vi "Parse State Queue++.vi"(0 "State Queue":string, 1 "Name(\"\" to use uuid)":string, 2 "Response Arguments":string, 7 "Error In (no error)":errorcluster, 9 "Dequeue Timeout(0ms)":i32, 11 "Response Timeout(1000ms)":i32=10000) -> (4 "Remaining States":string, 6 "Current State":string, 8 "Arguments":string, 10 "Argument - State":string, 15 "From Who":string)   [LabVIEW 2014, in "JKI-State-Machine-Plus.lvlib"]
doc: "Parses the JKI State Machine state queue and returns the current state that will execute next with the associated arguments.\n\nFor instructions on how to use the JKI State Machine, examples and video tutorials, visit:\nhttp://jkisoft.com/state-machine/\n\n<B>Inputs:</B>\n <B>State Queue:</B> The entire state queue is wired to this input. This should come from the main JKI State Machine shift register.\n <B>Error In</B> The error cluster from the JKI State Machine is wired to this input. If an error occures and appears on this input, the current state output returns the \"Error Handler\" state.\n\n<B>Outputs:</B>\n <B>Remaining States:</B> Returns all the next states that should execute after the current state completes. These should be passed through the current state in the state machine. These can also be modified or augmented within the current state if necessary.\n <B>Current State:</B> Returns the current state that should execute next in the state machine. If an error is wired to the Error input then the current state output becomes \"Error Handler\".\n <B>Arguments:</B> Returns any argument(s) that may be used in the current state string. These arguments come after the \">>\" characters. <B>Note:</B> The arguments variable must not contain any unprintable characters like linefeed or carriage return.\n\n<B>State Syntax:</B>\nStateCategory: State >> Argument\nLine Terminator: Line feed\n <B>Example:</B>\nUI: Help >> About\n\nWhere \"UI\" is the state category\nWhere \"Help\" is the state\nWhere \"About\" is the argument\n <B>Other Examples:</B>\nApp Data: Initialize\nUI: Initialize\nHelp >> About\n\n<B>Commenting:</B>\nTo add a comment use \"//\" or \"#\" and all text to the right will be ignored\n <B>Commenting Example:</B>\nUI: Initialize // This initializes the UI\n# This whole line is a comment\n// Another comment line\n\nJKI State Machine™ 2018.0.7.45\nhttp://jki.net/state-machine/\nCopyright (C) 2005-2018, JKI <info@jki.net>\nALL RIGHTS RESERVED"
uses:
  JKI-State-Machine-Plus.lvlib
  _Support/_Cross JKI StateMachine State Data.ctl
  _Support/_Cross JKI StateMachine State Response.ctl
  <vilib>/addons/_JKI Toolkits/State Machine/_JKI_lib_State_Machine.llb/Add State(s) to Queue__JKI_lib_State_Machine.vi
  Utility/Build Internal State String.vi
  _Support/_uuid.vi
  _Support/_JKISMQFGV.vi
  <vilib>/regexp/Match Regular Expression.xnode
panel:
  # "For instructions on how to use the JKI State Machine, examples and video tutorials, visit:\nhttp://jki.net/state-machine/\n\nJKI State Machine™\nhttp://jki.net/state-machine/\nCopyright (C) 2005-2017, JKI <info@jki.net>\nALL RIGHTS RESERVED"
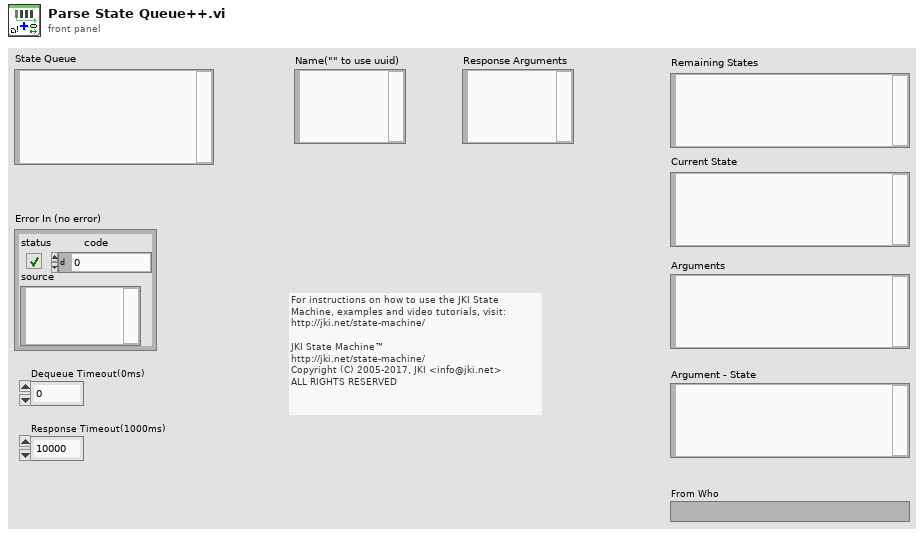
[diagram p1: front panel]
types:
  T1 = typedef "JKI-State-Machine-Plus.lvlib/_Cross JKI StateMachine State Data.ctl" = cluster{"state":string, "args":string, "source":string, "RespQ":refnum<queue>}
  T2 = typedef "JKI-State-Machine-Plus.lvlib/_Cross JKI StateMachine State Response.ctl" = cluster{"error":errorcluster, "Response Data":string}
  T3 = typedef "JKI-State-Machine-Plus.lvlib/_JKISMQ.ctl" = cluster{"Queue":refnum<queue>, "Locked Status":refnum<data-value>, "Stand Alone Mode":bool}
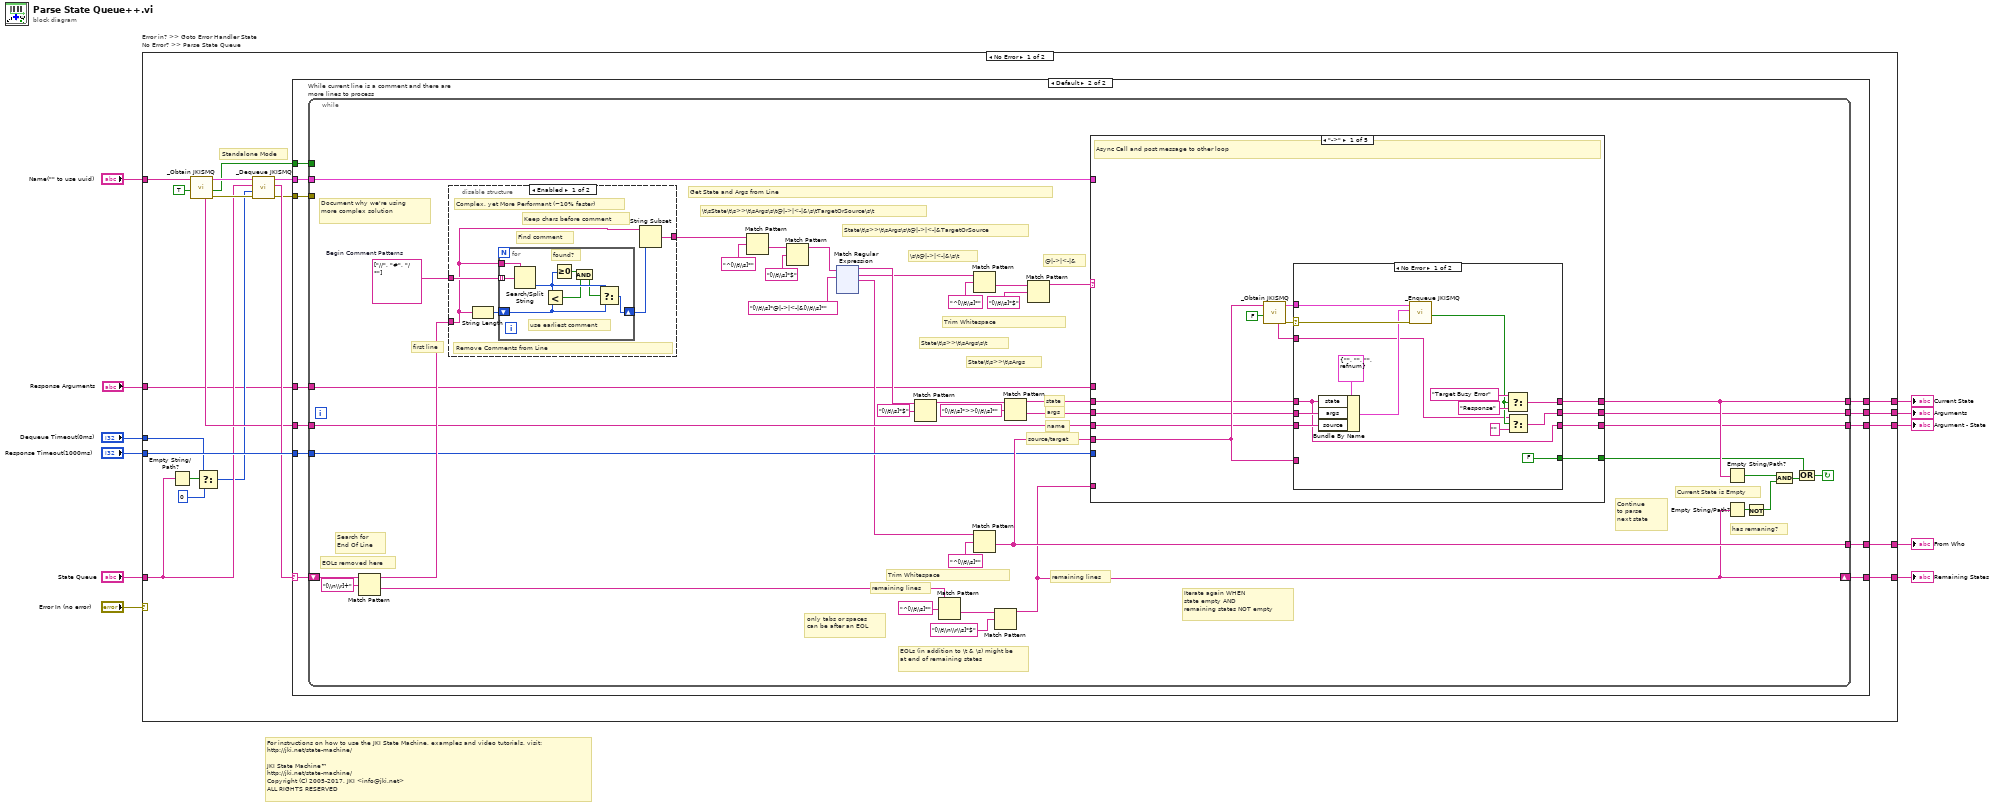
[diagram p0: block diagram]
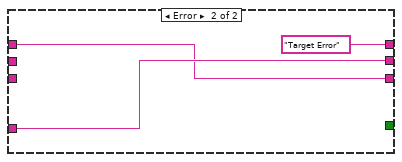
[diagram p3: hidden frame]
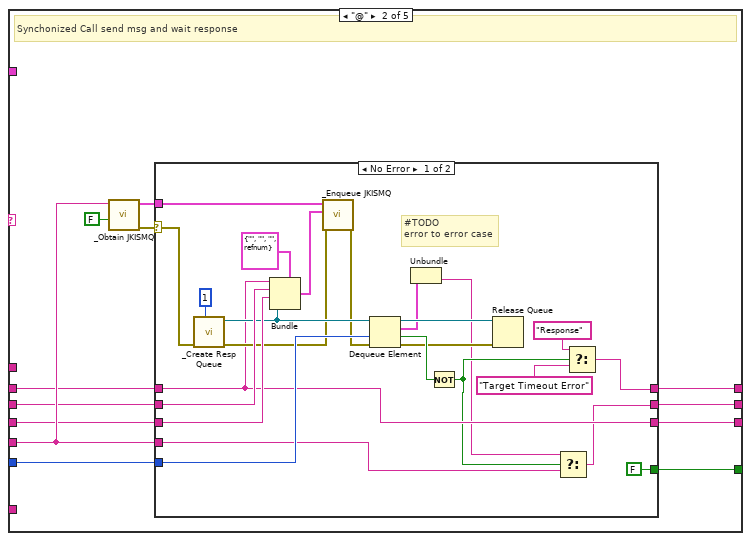
[diagram p4: hidden frame]
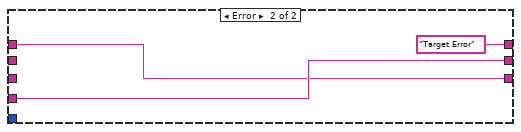
[diagram p5: hidden frame]
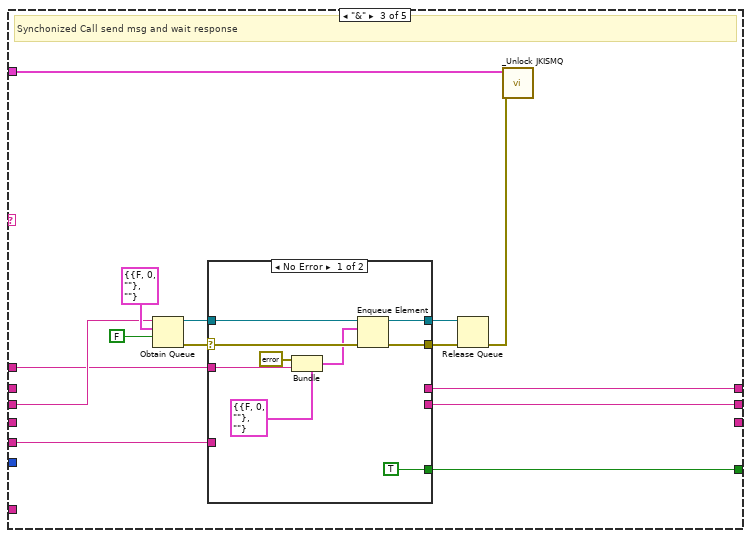
[diagram p6: hidden frame]
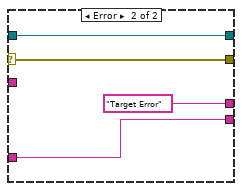
[diagram p7: hidden frame]
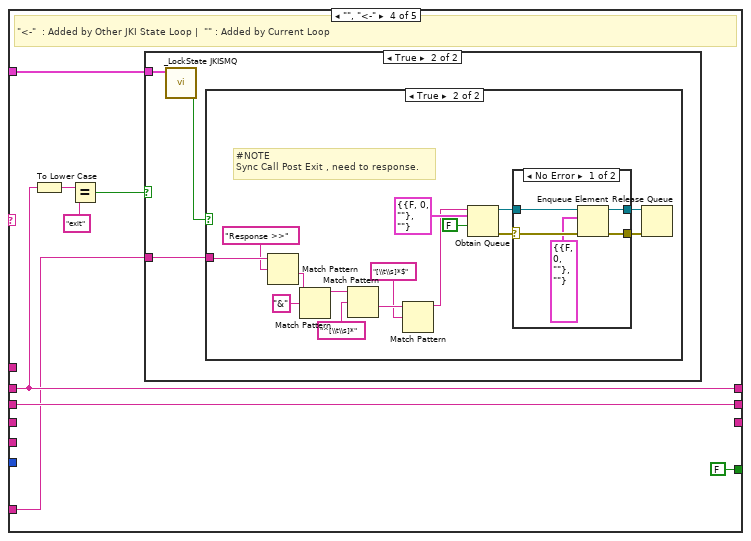
[diagram p8: hidden frame]
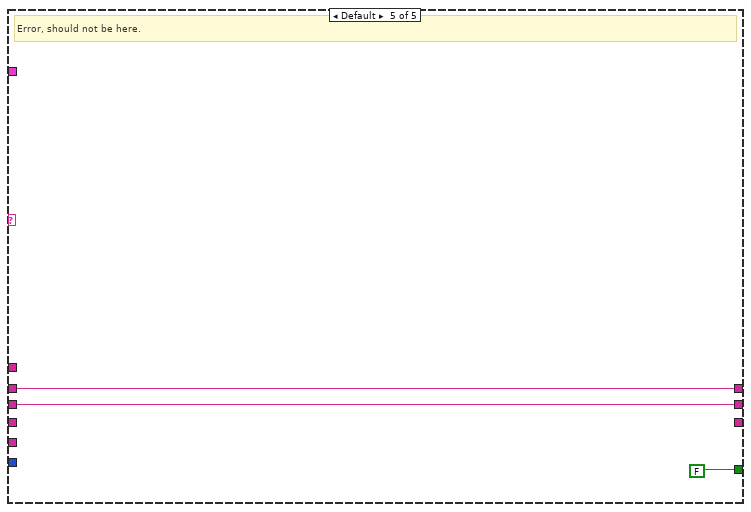
[diagram p12: hidden frame]
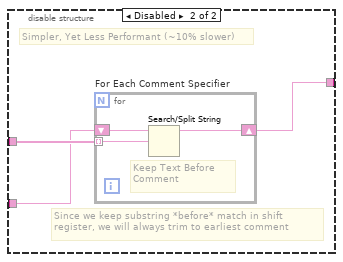
[diagram p13: hidden frame]
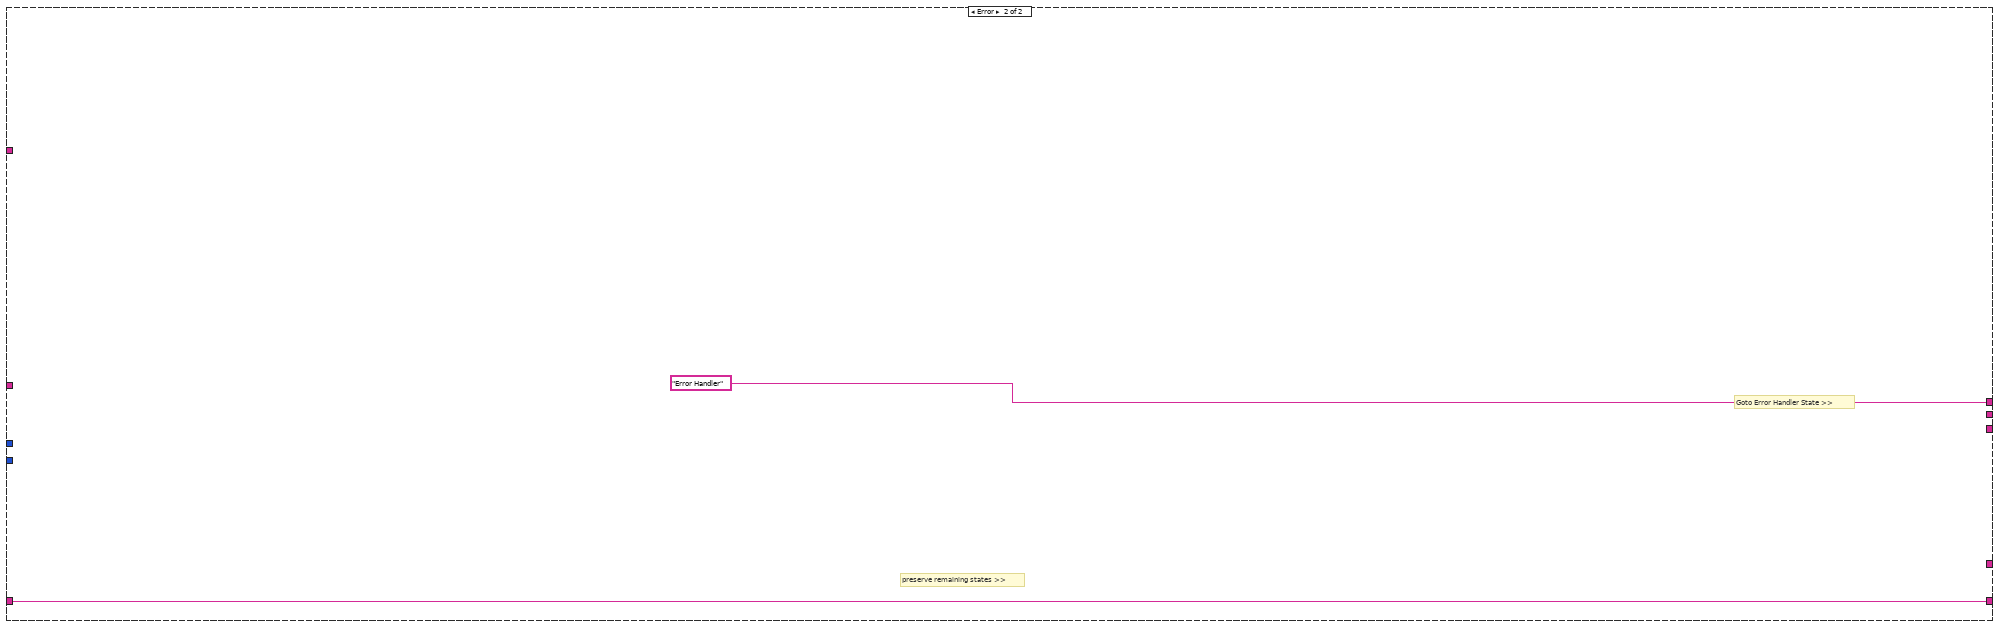
[diagram p14: hidden frame]
diagram:
  # "For instructions on how to use the JKI State Machine, examples and video tutorials, visit:\nhttp://jki.net/state-machine/\n\nJKI State Machine™\nhttp://jki.net/state-machine/\nCopyright (C) 2005-2017, JKI <info@jki.net>\nALL RIGHTS RESERVED"
  n1 = case "Error in? >> Goto Error Handler State\nNo Error? >> Parse State Queue" shown="No Error" "Error In (no error)" {
    tunnel: [w30 w353] -> w11
    tunnel: [w32 "Error Handler"] -> w9
    tunnel: [w31 _] -> w8
    tunnel: "State Queue" -> [w18 w353]
    tunnel: "Response Timeout(1000ms)" -> [w29 _]
    tunnel: "Name(\"\" to use uuid)" -> [w28 _]
    tunnel: [w27 _] -> w4
    tunnel: "Dequeue Timeout(0ms)" -> [w17 _]
    tunnel: [w13 _] -> w2
    tunnel: "Response Arguments" -> [w12 _]
    frame No Error {
      # "Standalone Mode"
      n2 = Empty String/Path?(string/path=w18) -> (empty?=w19:bool)
      n3 = call "_Obtain JKISMQ.vi"("create if not found? (T)"=TRUE, "Name(\"\" to use uuid) in"=w28) -> ("Error out"=w24:errorcluster, "Stand Alone Mode"=w14:bool, "JKISMQ"=w26:T3, "Name"=w21:string)  [unwired: 6 in]
      n4 = Select(t=w17, s=w19, f=0) -> (s? t:f=w15:i32)
      n5 = call "_Dequeue JKISMQ.vi"("Error in"=w24, "Dequeue Timeout(0ms)"=w15, "State(s) in (\"\")"=w18, "JKISMQ"=w26) -> ("Error out"=w20:errorcluster, "States Out"=w22:string, "JKISMQ"=w23:T3)  [unwired: 5 in]
      n6 = case shown="Default" w22 {
        selector: w22 -> [_ w38]
        tunnel: [_ w44] -> w32
        tunnel: [_ w43] -> w31
        tunnel: [_ w42] -> w30
        tunnel: w29 -> [_ w41]
        tunnel: [_ w40] -> w27
        tunnel: w21 -> [_ w39]
        tunnel: w23 -> [_ w37]
        tunnel: w20 -> [_ w36]
        tunnel: w14 -> [_ w35]
        tunnel: [_ w34] -> w13
        tunnel: w12 -> [_ w33]
        frame "" {
          # "Do Nothing if Empty String"
          # "<< Wiring into the Case Selector is much more performant than using \"Empty String/Path?\" primitive"
        }
        frame Default {
          n7 = while "While current line is a comment and there are more lines to process" {
            tunnel: [w77] -> w44
            tunnel: [w76] -> w43
            shift-right: [w68] -> w42
            shift-left: w38 -> [w83]
            tunnel: w41 -> [w70]
            tunnel: w39 -> [w75]
            tunnel: [w74] -> w40
            tunnel: w37 -> [w69]
            tunnel: w36 -> [_]
            tunnel: w35 -> [_]
            tunnel: [w46] -> w34
            tunnel: w33 -> [w45]
            stop <- w73 continue-if-true
            w82 = string[] ["//", "#", "/*"]  # Begin Comment Patterns
            # "Continue\nto parse \nnext state"
            # "source/target"
            # "name"
            # "@|->|<-|&"
            # "\\s\\t@|->|<-|&\\s\\t"
            # "Trim Whitespace"
            # "State\\t\\s>>\\t\\sArgs"
            # "State\\t\\s>>\\t\\sArgs\\s\\t"
            # "Get State and Args from Line"
            # "State\\t\\s>>\\t\\sArgs\\s\\t@|->|<-|&TargetOrSource"
            # "\\t\\sState\\t\\s>>\\t\\sArgs\\s\\t@|->|<-|&\\s\\tTargetOrSource\\s\\t"
            # "remaining lines"
            # "EOLs (in addition to \\t & \\s) might be at end of remaining states"
            # "Trim Whitespace"
            # "only tabs or spaces can be after an EOL"
            # "remaining lines"
            # "Iterate again WHEN\nstate empty AND\nremaining states NOT empty"
            # "args"
            # "state"
            # "Document why we're using more complex solution"
            # "EOLs removed here"
            # "Current State is Empty"
            # "has remaning?"
            # "first line"
            # "Search for End Of Line"
            n8 = Match Pattern(string=w83, regular expression="[\\n\\r]+") -> (before substring=w80:string, after substring=w78:string)  [unwired: 1 in, 2 out]
            n9 = disable-structure "Diagram Disable Structure" shown="Enabled" {
              disable-tunnel: w82 -> [w337 w348]
              disable-tunnel: [w336 w347] -> w81
              disable-tunnel: w80 -> [w335 w346]
              frame Enabled {
                # "Remove Comments from Line"
                # "Complex, yet More Performant (~10% faster)"
                # "Keep chars before comment"
                # "Find comment"
                n10 = String Length(string=w335) -> (length=w334:i32)
                n11 = for {
                  tunnel: w337 -> [w342] mode=indexing
                  shift-right: [w344] -> w333
                  shift-left: w334 -> [w345]
                  tunnel: w335 -> [w343]
                  # "found?"
                  # "use earliest comment"
                  n12 = Search/Split String(string=w343, search string/char (-)=w342) -> (offset of match=w341:i32)  [unwired: 1 in, 2 out]
                  n13 = Less?(x=w341, y=w345) -> (x < y?=w339:bool)
                  n14 = Greater Or Equal To 0?(x=w341) -> (x >= 0?=w340:bool)
                  n15 = And(x=w340, y=w339) -> (x .and. y?=w338:bool)
                  n16 = Select(t=w341, s=w338, f=w345) -> (s? t:f=w344:i32)
                }
                n17 = String Subset(string=w335, length (rest)=w333) -> (substring=w336:string)  [unwired: 1 in]
              }
              frame Disabled {
                # "Since we keep substring *before* match in shift register, we will always trim to earliest comment"
                # "Simpler, Yet Less Performant (~10% slower)"
                n18 = for "For Each Comment Specifier" {
                  tunnel: w348 -> [w350] mode=indexing
                  shift-right: [w349] -> w347
                  shift-left: w346 -> [w351]
                  # "Keep Text Before Comment"
                  n19 = Search/Split String(string=w351, search string/char (-)=w350) -> (substring before match=w349:string)  [unwired: 1 in, 2 out]
                }
              }
            }
            n20 = Match Pattern(string=w81, regular expression="^[\\t\\s]*") -> (after substring=w61:string)  [unwired: 1 in, 3 out]
            n21 = Match Pattern(string=w61, regular expression="[\\t\\s]*$") -> (before substring=w47:string)  [unwired: 1 in, 3 out]
            n22 = xnode "Match Regular Expression"("input string"=w47, "regular expression"="[\\t\\s]*@|->|<-|&[\\t\\s]*") -> ("before match"=w58:string, "whole match"=w55:string, "after match"=w48:string)  [unwired: 4 in, 2 out]
            n23 = Match Pattern(string=w58, regular expression="[\\t\\s]*$") -> (before substring=w57:string)  [unwired: 1 in, 3 out]
            n24 = Match Pattern(string=w78, regular expression="^[\\t\\s]*") -> (after substring=w62:string)  [unwired: 1 in, 3 out]
            n25 = Match Pattern(string=w55, regular expression="^[\\t\\s]*") -> (after substring=w51:string)  [unwired: 1 in, 3 out]
            n26 = Match Pattern(string=w48, regular expression="^[\\t\\s]*") -> (after substring=w74:string)  [unwired: 1 in, 3 out]
            n27 = Match Pattern(string=w62, regular expression="[\\t\\n\\r\\s]*$") -> (before substring=w68:string)  [unwired: 1 in, 3 out]
            n28 = Match Pattern(string=w57, regular expression="[\\t\\s]*>>[\\t\\s]*") -> (before substring=w54:string, after substring=w53:string)  [unwired: 1 in, 2 out]
            n29 = Match Pattern(string=w51, regular expression="[\\t\\s]*$") -> (before substring=w50:string)  [unwired: 1 in, 3 out]
            n30 = case shown="\"->\"" w50 {
              tunnel: w54 -> [w91 w120 _ w188 w218]
              tunnel: w53 -> [w90 w119 w159 w190 w217]
              tunnel: [w97 w126 w168 w188 w218] -> w77
              tunnel: [w96 w125 w167 w190 w217] -> w76
              tunnel: w75 -> [w89 w118 _ _ _]
              tunnel: w74 -> [w94 w124 w160 _ _]
              tunnel: [w98 w127 w169 FALSE FALSE] -> w71
              tunnel: w70 -> [_ w128 _ _ _]
              tunnel: w69 -> [_ _ w158 w183 _]
              tunnel: w68 -> [_ _ _ w185 _]
              tunnel: [w87 w117 _ _ _] -> w46
              tunnel: w45 -> [_ _ w156 _ _]
              frame "->" {
                # "Async Call and post message to other loop"
                n31 = call "_Obtain JKISMQ.vi"("create if not found? (T)"=FALSE, "Name(\"\" to use uuid) in"=w94) -> ("Error out"=w92:errorcluster, "JKISMQ"=w93:T3, "Name"=w88:string)  [unwired: 6 in, 1 out]
                n32 = case shown="No Error" w92 {
                  selector: w92 -> [w112 _]
                  tunnel: w93 -> [w113 _]
                  tunnel: [FALSE _] -> w98
                  tunnel: [w104 "Target Error" ("before match")] -> w97
                  tunnel: [w100 w115] -> w96
                  tunnel: w94 -> [_ w115]
                  tunnel: w91 -> [w99 w114]
                  tunnel: w90 -> [w109 _]
                  tunnel: w89 -> [w108 _]
                  tunnel: w88 -> [w101 _]
                  tunnel: [w99 w114] -> w87
                  frame No Error {
                    n33 = Bundle By Name(cluster=T1 {"state"="", "args"="", "source"="", "RespQ"=refnum} ("Cross JKI State Machine State"), "state"=w99, "args"=w109, "source"=w108) -> (w107:T1)
                    n34 = call "_Enqueue JKISMQ.vi"("Error in"=w112, "Data"=w107, "JKISMQ"=w113) -> ("Target Buzy Error"=w102:bool)  [unwired: 6 in, 2 out]
                    n35 = Select(t="Target Buzy Error" ("f"), s=w102, f="Response" ("before match")) -> (s? t:f=w104:string)
                    n36 = Select(t=w101, s=w102, f="" ("before match")) -> (s? t:f=w100:string)
                  }
                  frame Error {
                  }
                }
              }
              frame "@" {
                # "Synchonized Call send msg and wait response"
                n37 = call "_Obtain JKISMQ.vi"("create if not found? (T)"=FALSE, "Name(\"\" to use uuid) in"=w124) -> ("Error out"=w122:errorcluster, "JKISMQ"=w123:T3)  [unwired: 6 in, 2 out]
                n38 = case shown="No Error" w122 {
                  selector: w122 -> [w140 _]
                  tunnel: w128 -> [w151 _]
                  tunnel: w123 -> [w152 _]
                  tunnel: [FALSE _] -> w127
                  tunnel: [w150 "Target Error" ("before match")] -> w126
                  tunnel: [w129 w154] -> w125
                  tunnel: w124 -> [w130 w154]
                  tunnel: w120 -> [w134 w153]
                  tunnel: w119 -> [w145 _]
                  tunnel: w118 -> [w144 _]
                  tunnel: [w134 w153] -> w117
                  frame No Error {
                    # "#TODO \nerror to error case"
                    n39 = call "_Create Resp Queue.vi"("max queue size (-1, unlimited)"=1, "error in (no error)"=w140) -> ("error out"=w136:errorcluster, "queue out"=w141:refnum<queue>)  [unwired: 7 in, 1 out]
                    n40 = Bundle(cluster=T1 {"state"="", "args"="", "source"="", "RespQ"=refnum} ("Cross JKI State Machine State"), "state"=w134, "args"=w145, "source"=w144, "RespQ"=w141) -> (w142:T1)
                    n41 = call "_Enqueue JKISMQ.vi"("Error in"=w136, "Data"=w142, "JKISMQ"=w152) -> ("Error out"=w137:errorcluster)  [unwired: 6 in, 2 out]
                    n42 = Dequeue Element(queue=w141, timeout in ms (-1)=w151, error in (no error)=w137) -> (queue out=w139:refnum<queue>, element=w135:T2, timed out?=w149:bool, error out=w138:errorcluster)
                    n43 = Unbundle(w135) -> ("Response Data"=w131:string)  [unwired: 1 out]
                    n44 = Not(x=w149) -> (.not. x?=w132:bool)
                    n45 = Release Queue(queue=w139, error in (no error)=w138) -> ()  [unwired: 1 in, 3 out]
                    n46 = Select(t=w131, s=w132, f=w130) -> (s? t:f=w129:string)
                    n47 = Select(t="Response" ("f"), s=w132, f="Target Timeout Error" ("before match")) -> (s? t:f=w150:string)
                  }
                  frame Error {
                  }
                }
              }
              frame "&" {
                # "Synchonized Call send msg and wait response"
                n48 = Obtain Queue(name (unnamed)=w159, element data type=T2 {"error"={"status"=FALSE, "code"=0, "source"=""}, "Response Data"=""} ("Cross JKI State Machine Response"), create if not found? (T)=FALSE) -> (queue out=w164:refnum<queue>, error out=w163:errorcluster)  [unwired: 2 in, 1 out]
                n49 = case shown="No Error" w163 {
                  selector: w163 -> [w176 w180]
                  tunnel: [TRUE _] -> w169
                  tunnel: [_ "Target Error" ("before match")] -> w168
                  tunnel: [_ w179] -> w167
                  tunnel: w164 -> [w178 w181]
                  tunnel: [w177 w181] -> w166
                  tunnel: [w175 w180] -> w165
                  tunnel: w160 -> [_ w179]
                  tunnel: w156 -> [w171 _]
                  frame No Error {
                    n50 = Bundle(cluster=T2 {"error"={"status"=FALSE, "code"=0, "source"=""}, "Response Data"=""} ("element"), "error"=errorcluster {"status"=FALSE, "code"=0, "source"=""}, "Response Data"=w171) -> (w172:T2)
                    n51 = Enqueue Element(queue=w178, element=w172, error in (no error)=w176) -> (queue out=w177:refnum<queue>, error out=w175:errorcluster)  [unwired: 1 in, 1 out]
                  }
                  frame Error {
                  }
                }
                n52 = Release Queue(queue=w166, error in (no error)=w165) -> (error out=w157:errorcluster)  [unwired: 1 in, 2 out]
                n53 = call "_Unlock JKISMQ.vi"("Error in"=w157, "JKISMQ"=w158) -> ()  [unwired: 8 in, 2 out]
              }
              frame "", "<-" {
                # "\"<-\"  : Added by Other JKI State Loop |  \"\" : Added by Current Loop"
                n54 = To Lower Case(string=w188) -> (all lower case string=w187:string)
                n55 = Equal?(x=w187, y="exit") -> (x = y?=w184:bool)
                n56 = case shown="True" w184 {
                  tunnel: w185 -> [_ w193]
                  tunnel: w183 -> [_ w192]
                  frame False {
                  }
                  frame True {
                    n57 = call "_LockState JKISMQ.vi"("JKISMQ"=w192) -> ("lock"=w191:bool)  [unwired: 8 in, 2 out]
                    n58 = case shown="True" w191 {
                      tunnel: w193 -> [_ w202]
                      frame False {
                      }
                      frame True {
                        # "#NOTE\nSync Call Post Exit , need to response."
                        n59 = Match Pattern(string=w202, regular expression="Response >>") -> (after substring=w199:string)  [unwired: 1 in, 3 out]
                        n60 = Match Pattern(string=w199, regular expression="&") -> (before substring=w195:string)  [unwired: 1 in, 3 out]
                        n61 = Match Pattern(string=w195, regular expression="^[\\t\\s]*") -> (after substring=w198:string)  [unwired: 1 in, 3 out]
                        n62 = Match Pattern(string=w198, regular expression="[\\t\\s]*$") -> (before substring=w194:string)  [unwired: 1 in, 3 out]
                        n63 = Obtain Queue(name (unnamed)=w194, element data type=T2 {"error"={"status"=FALSE, "code"=0, "source"=""}, "Response Data"=""} ("Cross JKI State Machine Response"), create if not found? (T)=FALSE) -> (queue out=w207:refnum<queue>, error out=w208:errorcluster)  [unwired: 2 in, 1 out]
                        n64 = case shown="No Error" w208 {
                          selector: w208 -> [w211 w214]
                          tunnel: w207 -> [w213 w215]
                          tunnel: [w212 w215] -> w205
                          tunnel: [w210 w214] -> w206
                          frame No Error {
                            n65 = Enqueue Element(queue=w213, element=T2 {"error"={"status"=FALSE, "code"=0, "source"=""}, "Response Data"=""}, error in (no error)=w211) -> (queue out=w212:refnum<queue>, error out=w210:errorcluster)  [unwired: 1 in, 1 out]
                          }
                          frame Error {
                          }
                        }
                        n66 = Release Queue(queue=w205, error in (no error)=w206) -> ()  [unwired: 1 in, 3 out]
                      }
                    }
                  }
                }
              }
              frame Default {
                # "Error, should not be here."
              }
            }
            n67 = Empty String/Path?(string/path=w77) -> (empty?=w86:bool)
            n68 = Empty String/Path?(string/path=w68) -> (empty?=w85:bool)
            n69 = Not(x=w85) -> (.not. x?=w79:bool)
            n70 = And(x=w86, y=w79) -> (x .and. y?=w72:bool)
            n71 = Or(x=w71, y=w72) -> (x .or. y?=w73:bool)
          }
        }
      }
    }
    frame Error {
      # "Goto Error Handler State >>"
      # "preserve remaining states >>"
    }
  }
  "Remaining States" <- w11
  "Arguments" <- w8
  "Current State" <- w9
  "From Who" <- w4
  "Argument - State" <- w2
